vi "Wzmacniacz.vi"(4 "Milisekund_na_dane":u32, 6 "Rodzaj_wzmacniacza":T1, 7 "Wartosc_poprzednia":dbl, 9 "Wzmocnienie":dbl, 10 "Parametry_cosinusow":T2, 11 "Czas":dbl) -> (2 "Wartosc_poprzednia":dbl, 3 "Sygnal_wzmocniony":dbl)   [LabVIEW 2020]
doc: "VI zwraca wartosci wzmocnionego sygnalu modulujacego"
uses:
  Kontrolki/Parametry_cosinusow.ctl
  Kontrolki/Parametry_cosinusa.ctl
  Kontrolki/Rodzaj_wzmacniacza.ctl
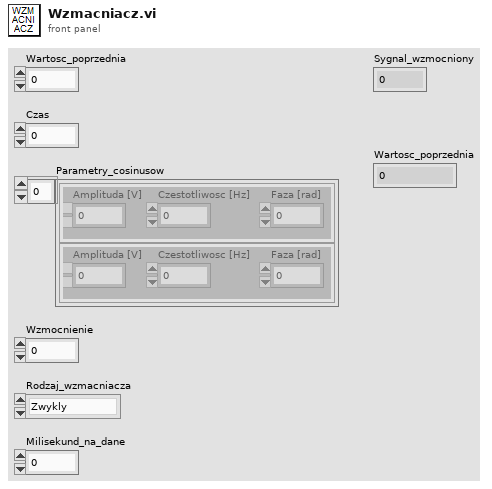
[diagram p1: front panel]
types:
  T1 = typedef "Rodzaj_wzmacniacza.ctl" = enum16{"Zwykly", "Calkujacy", "Rozniczkujacy"}
  T2 = typedef "Parametry_cosinusow.ctl" = T3[]
  T3 = typedef "Parametry_cosinusa.ctl" = cluster{"Amplituda [V]":dbl, "Czestotliwosc [Hz] ":dbl, "Faza [rad]":dbl}
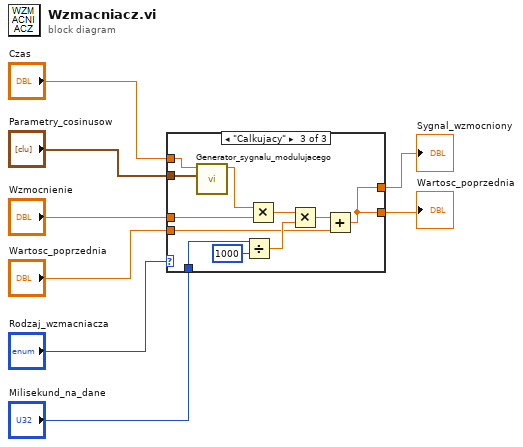
[diagram p0: block diagram]
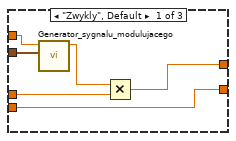
[diagram p2: hidden frame]
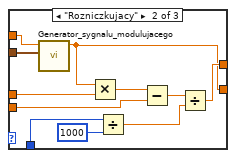
[diagram p3: hidden frame]
diagram:
  n1 = case shown="\"Calkujacy\"" "Rodzaj_wzmacniacza" {
    tunnel: "Parametry_cosinusow" -> [w14 w25 w36]
    tunnel: "Czas" -> [w13 w24 w35]
    tunnel: "Wzmocnienie" -> [w11 w23 w33]
    tunnel: [w9 w15 w26] -> w5
    tunnel: "Wartosc_poprzednia" -> [w9 w22 w27]
    tunnel: [w10 w17 w26] -> w7
    tunnel: "Milisekund_na_dane" -> [_ w20 w32]
    frame "Zwykly", Default {
      n2 = call "Generator_sygnalu_modulujacego.vi"("Parametry_cosinusow"=w14, "Czas"=w13) -> ("Sygnal_modulujacy"=w12:dbl)  [unwired: 9 in]
      n3 = Multiply(x=w12, y=w11) -> (x*y=w10:dbl)
    }
    frame "Rozniczkujacy" {
      n4 = call "Generator_sygnalu_modulujacego.vi"("Parametry_cosinusow"=w25, "Czas"=w24) -> ("Sygnal_modulujacy"=w15:dbl)  [unwired: 9 in]
      n5 = Multiply(x=w15, y=w23) -> (x*y=w21:dbl)
      n6 = Divide(x=w20, y=1000) -> (x/y=w16:dbl)
      n7 = Subtract(x=w21, y=w22) -> (x-y=w18:dbl)
      n8 = Divide(x=w18, y=w16) -> (x/y=w17:dbl)
    }
    frame "Calkujacy" {
      n9 = call "Generator_sygnalu_modulujacego.vi"("Parametry_cosinusow"=w36, "Czas"=w35) -> ("Sygnal_modulujacy"=w34:dbl)  [unwired: 9 in]
      n10 = Divide(x=w32, y=1000) -> (x/y=w29:dbl)
      n11 = Multiply(x=w34, y=w33) -> (x*y=w30:dbl)
      n12 = Multiply(x=w30, y=w29) -> (x*y=w28:dbl)
      n13 = Add(x=w28, y=w27) -> (x+y=w26:dbl)
    }
  }
  "Sygnal_wzmocniony" <- w7
  "Wartosc_poprzednia" <- w5
